vi "Event Handler.vi"(8 "error in (no error)":errorcluster, 10 "Stop Event Handler":refnum<user-event>, 11 "SliderBG in":refnum<class "SlideBackgroundGradient.lvclass">) -> (0 "error out":errorcluster)   [LabVIEW 2015, in "SlideBackgroundGradient.lvclass"]
doc: "The <b>Event Handler VI</b> is a dynamic dispatch VI that should be overwritten if events are needed to create the enhanced QControl. \n\nBy inheriting from the main Control.lvclass the overwritten <b>Event Handler VI</b> will be launched asynchronously in the initialization of the QControl.\n<b> </b> <b> </b>\n©2016 Q Software Innovations, LLC (QSI)\nwritten by Quentin Alldredge\nproduced in LabVIEW 2015\n\nsupport@qsoftwareinnovations.com\nwww.qsoftwareinnovations.com\n\nAll rights reserved.\n\nRedistribution and use in source and binary forms, with or without modification, are permitted provided that the following conditions are met:\n\n * Redistributions of source code must retain the above copyright notice, this list of conditions and the following disclaimer.\n * Redistributions in binary form must reproduce the above copyright notice, this list of conditions and the following disclaimer in the documentation and/or other materials provided with the distribution.\n * Neither the name of Q Software Innovations, LLC. nor the names of its contributors may be used to endorse or promote products derived from this software without specific prior written permission.\n\nTHIS SOFTWARE IS PROVIDED BY THE COPYRIGHT HOLDERS AND CONTRIBUTORS \"AS IS\" AND ANY EXPRESS OR IMPLIED WARRANTIES, INCLUDING, BUT NOT LIMITED TO, THE IMPLIED WARRANTIES OF MERCHANTABILITY AND FITNESS FOR A PARTICULAR PURPOSE ARE DISCLAIMED. IN NO EVENT SHALL THE COPYRIGHT OWNER OR CONTRIBUTORS BE LIABLE FOR ANY DIRECT, INDIRECT, INCIDENTAL, SPECIAL, EXEMPLARY, OR CONSEQUENTIAL DAMAGES (INCLUDING, BUT NOT LIMITED TO, PROCUREMENT OF SUBSTITUTE GOODS OR SERVICES; LOSS OF USE, DATA, OR PROFITS; OR BUSINESS INTERRUPTION) HOWEVER CAUSED AND ON ANY THEORY OF LIABILITY, WHETHER IN CONTRACT, STRICT LIABILITY, OR TORT (INCLUDING NEGLIGENCE OR OTHERWISE) ARISING IN ANY WAY OUT OF THE USE OF THIS SOFTWARE, EVEN IF ADVISED OF THE POSSIBILITY OF SUCH DAMAGE."
uses:
  SlideBackgroundGradient.lvclass
  SlideBackgroundGradient.lvclass/SlideBackgroundGradient.ctl
  Read StartColor.vi
  Read EndColor.vi
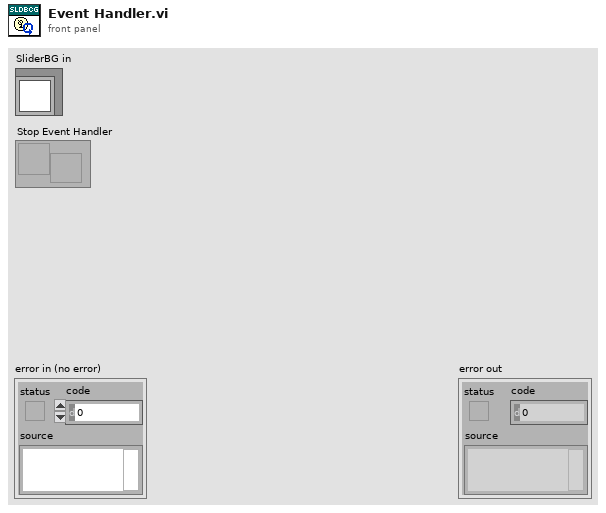
[diagram p1: front panel]
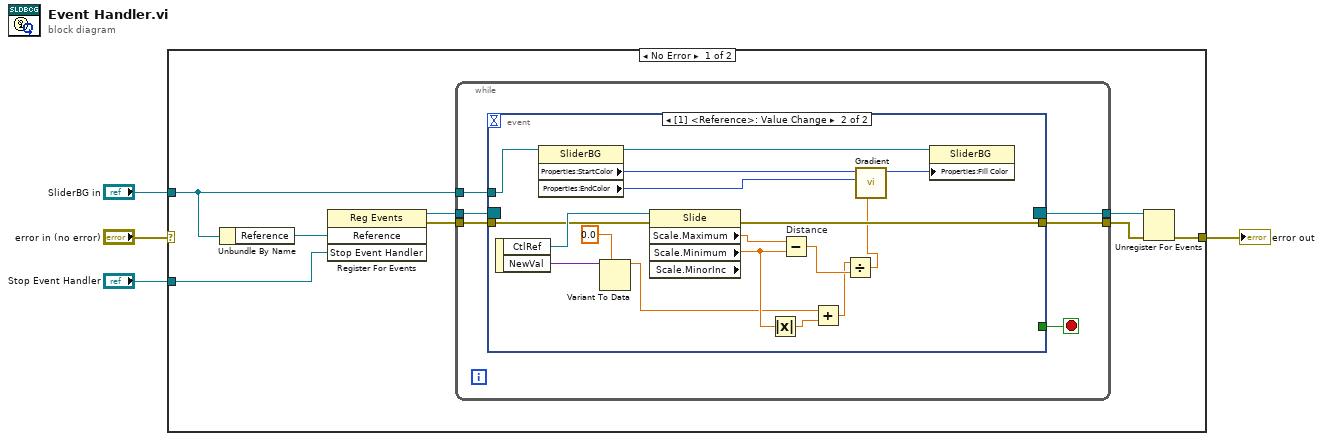
[diagram p0: block diagram]
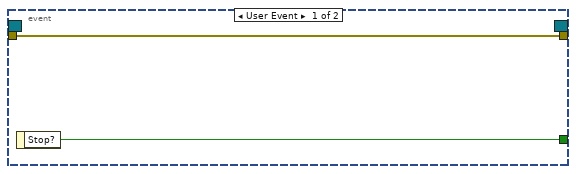
[diagram p2: hidden frame]
diagram:
  n1 = case shown="No Error" "error in (no error)" {
    selector: "error in (no error)" -> [_ w38]
    tunnel: [w8 w38] -> w3
    tunnel: "SliderBG in" -> [w7 _]
    tunnel: "Stop Event Handler" -> [w5 _]
    frame No Error {
      n2 = Unbundle By Name(w7) -> ("Reference"=w6:refnum<vi>)
      n3 = register-events(w6, w5) -> (reference out=w12:refnum<event-registration>, error out=w11:errorcluster)  [unwired: 2 in]
      n4 = while {
        tunnel: w12 -> [w17]
        tunnel: w11 -> [w16]
        tunnel: [w14] -> w10
        tunnel: [w13] -> w9
        tunnel: w7 -> [w18]
        stop <- w15 stop-if-true
        n5 = event shown="[1] <Reference>: Value Change" {
          selector: w17 -> [_ _]
          dyn-events: [_ _] -> w14
          timeout: _ -> [_ _]
          tunnel: w18 -> [_ w30]
          tunnel: w16 -> [w19 w34]
          tunnel: [w20 _] -> w15
          tunnel: [w19 w33] -> w13
          event User Event {
            n6 = event-data() -> ("Stop?"=w20:bool)  [unwired: 1 in]
          }
          event Value Change {
            n7 = event-data() -> ("CtlRef"=w35:refnum<vi>, "NewVal"=w37:variant)  [unwired: 1 in]
            n8 = property class="SliderBG"(reference=w30) -> (reference out=w25:refnum<class "SlideBackgroundGradient.lvclass">, "Properties:StartColor"=w21:u32, "Properties:EndColor"=w22:u32)  [unwired: 1 in, 1 out]
            n9 = Variant To Data(type=0.0, Variant=w37) -> (data=w27:dbl)  [unwired: 1 in, 1 out]
            n10 = property class="Slide" props=["Scale", "Maximum", "Scale", "Minimum", "Scale", "MinorInc"](reference=w35, error in=w34) -> (error out=w33:errorcluster, "Scale.Maximum"=w32:dbl, "Scale.Minimum"=w29:dbl)  [unwired: 2 out]
            n11 = Absolute Value(x=w29) -> (abs(x)=w28:dbl)
            n12 = Subtract "Distance"(x=w32, y=w29) -> (x-y=w31:dbl)
            n13 = Add(x=w27, y=w28) -> (x+y=w26:dbl)
            n14 = Divide(x=w26, y=w31) -> (x/y=w23:dbl)
            n15 = call "Gradient.vi"("Percent"=w23, "End Color"=w22, "Start Color"=w21) -> ("Gradient Color"=w24:u32)  [unwired: 8 in]
            n16 = property class="SliderBG"(reference=w25, "Properties:Fill Color"=w24) -> ()  [unwired: 1 in, 2 out]
          }
        }
      }
      n17 = Unregister For Events(event registration refnum=w10, error in=w9) -> (error out=w8:errorcluster)
    }
    frame Error {
    }
  }
  "error out" <- w3
